vi "Demo.vi"() -> ()   [LabVIEW 2018, in "Cfg.lvlib"]
uses:
  Cfg.lvlib
  d3ed3220-b1c1-459d-aa1c-7c40294cb342.vi
  Operation.ctl
panel:
  out "Remove Section Found?":bool
  out "Remove Key Found?":bool
  out "All Sections":T1(array[cluster])
  out "Section Found?":bool
  out "Keys":string[](array[string])
  out "Sections":string[](array[string])
  out "error out":errorcluster
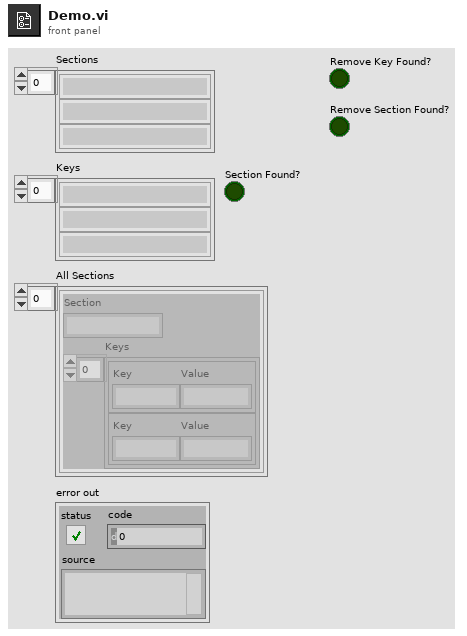
[diagram p1: front panel]
types:
  T1 = cluster{"Section":string, "Keys":cluster{"Key":string, "Value":string}[]}[]
  T2 = typedef "Cfg.lvlib/Operation.ctl" = enum8{"Read or Create", "Read", "Write"}
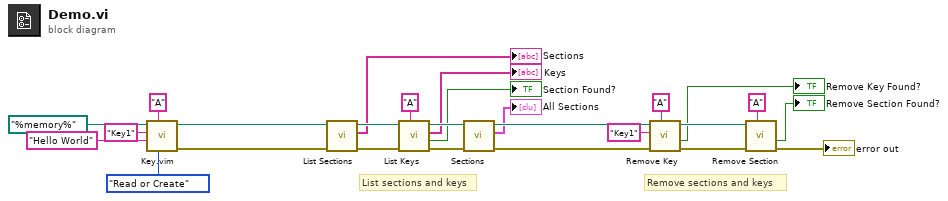
[diagram p0: block diagram]
diagram:
  # "Remove sections and keys"
  # "List sections and keys"
  n1 = call "Key.vim"("Operation (Read or Create)"=Operation."Read or Create", "Section"="A", "Value"="Hello World", "Key"="Key1", "Ini Path in"=path "%memory%") -> ("error out"=w7:errorcluster, "Ini Path out"=w8:path)  [unwired: 3 in, 2 out]
  n2 = call "List Sections.vi"("error in (no error)"=w7, "Ini Path in"=w8) -> ("error out"=w12:errorcluster, "Sections"=→"Sections":string[], "Ini Path out"=w11:path)  [unwired: 7 in]
  n3 = call "List Keys.vi"("Section"="A", "error in (no error)"=w12, "Ini Path in"=w11) -> ("error out"=w9:errorcluster, "Section Found?"=→"Section Found?":bool, "Keys"=→"Keys":string[], "Ini Path out"=w10:path)  [unwired: 5 in]
  n4 = call "Sections.vi"("error in (no error)"=w9, "Ini Path in"=w10) -> ("error out"=w18:errorcluster, "All Sections"=→"All Sections":T1, "Ini Path out"=w17:path)  [unwired: 7 in]
  n5 = call "Remove Key.vi"("Section"="A", "error in (no error)"=w18, "Key"="Key1", "Ini Path in"=w17) -> ("error out"=w25:errorcluster, "Key Found?"=→"Remove Key Found?":bool, "Ini Path out"=w24:path)  [unwired: 5 in]
  n6 = call "Remove Section.vi"("Section"="A", "error in (no error)"=w25, "Ini Path in"=w24) -> ("error out"=→"error out":errorcluster, "Section Found?"=→"Remove Section Found?":bool)  [unwired: 6 in, 1 out]
